vi "outer_vi.vi"() -> ()   [LabVIEW 2011]
panel:
  out "Value 2":bool
  in  "OK Button":bool
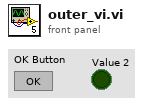
[diagram p1: front panel]
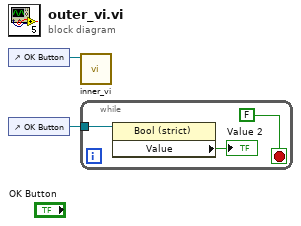
[diagram p0: block diagram]
diagram:
  n1 = control-ref of="OK Button"() -> (w1:refnum<vi>)
  n2 = control-ref of="OK Button"() -> (w2:refnum<vi>)
  n3 = call "inner_vi.vi"("Bool Refnum"=w1) -> ()  [unwired: 11 in]
  n4 = while {
    tunnel: w2 -> [w4]
    stop <- FALSE stop-if-true
    n5 = property class="Bool (strict)"(reference=w4) -> ("Value"=→"Value 2":bool)  [unwired: 1 in, 2 out]
  }
